vi "Preview.vi"(8 "error in (no error)":errorcluster, 11 "Password Protected VI Path":path) -> (0 "error out":errorcluster)   [LabVIEW 2021, in "VI-Hacker.lvlib"]
doc: "Unlock and preview a password protected VI."
uses:
  VI-Hacker.lvlib
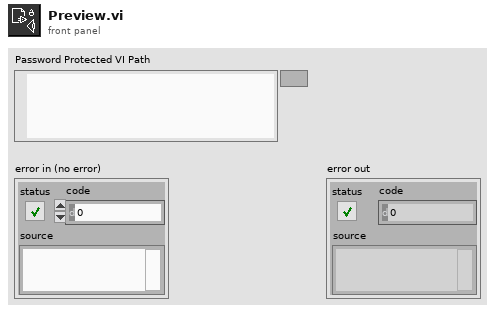
[diagram p1: front panel]
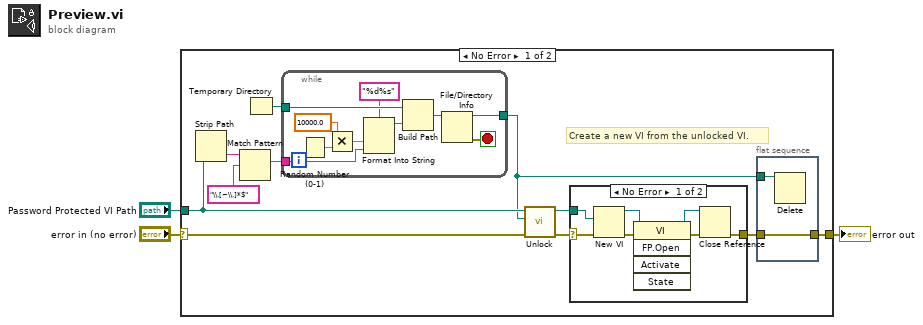
[diagram p0: block diagram]
diagram:
  n1 = case shown="No Error" "error in (no error)" {
    selector: "error in (no error)" -> [w10 w35]
    tunnel: "Password Protected VI Path" -> [w7 _]
    tunnel: [w5 w35] -> w1
    frame No Error {
      # "Create a new VI from the unlocked VI."
      n2 = Strip Path(path=w7) -> (name=w13:string)  [unwired: 1 out]
      n3 = Match Pattern(string=w13, regular expression="\\.[~\\.]*$") -> (match substring=w11:string)  [unwired: 4 out]
      n4 = Temporary Directory() -> (w14:path)
      n5 = while {
        tunnel: w14 -> [w34]
        tunnel: w11 -> [w26]
        tunnel: [w25] -> w6
        stop <- w32 stop-if-true
        n6 = Random Number (0-1)() -> (number: 0 to 1=w31:dbl)
        n7 = Multiply(x=10000.0, y=w31) -> (x*y=w29:dbl)
        n8 = Format Into String(format string="%d%s", w29, w26) -> (resulting string=w28:string)  [unwired: 2 in, 1 out]
        n9 = Build Path(base path=w34, name or relative path=w28) -> (appended path=w33:path)
        n10 = File/Directory Info(path=w33) -> (path out=w25:path, error out=w32:errorcluster)  [unwired: 1 in, 5 out]
      }
      n11 = call "Unlock.vi"("error in (no error)"=w10, "New VI Path"=w6, "Password Protected VI Path"=w7) -> ("error out"=w9:errorcluster, "Unlocked VI Path"=w8:path)  [unwired: 7 in]
      n12 = case shown="No Error" w9 {
        selector: w9 -> [w18 w24]
        tunnel: [w19 w24] -> w4
        tunnel: w8 -> [w17 _]
        frame No Error {
          n13 = New VI(8:w18, 10:w17) -> (0:w23:errorcluster, 3:w22:refnum<vi>)  [unwired: 5 in]
          n14 = invoke class="VI" method="FP.Open"(reference=w22, error in=w23) -> (reference out=w20:refnum<vi>, error out=w21:errorcluster)  [unwired: 3 in, 3 out]
          n15 = Close Reference(reference=w20, error in (no error)=w21) -> (error out=w19:errorcluster)
        }
        frame Error {
        }
      }
      n16 = flat-sequence {
        tunnel: w6 -> [w16]
        tunnel: [w15] -> w5
        tunnel: w4 -> [w15]
        frame #0 {
          n17 = Delete(path (use dialog)=w16) -> ()  [unwired: 4 in, 3 out]
        }
      }
    }
    frame Error {
    }
  }
  "error out" <- w1
